vi "Check LVAddons Path List.vi"() -> ()   [LabVIEW 2023]
uses:
  <vilib>/Utility/Symbolic Paths/NI_SymbolicPaths.lvlib
  <vilib>/Utility/Symbolic Paths/Symbolic Path ID--enum.ctl
panel:
  out "all resolved paths":path[](array[path])
  # "Run this VI and verify that your LVAddon development location is in the list of paths.\n\nIf not, verify the correct paths are in the custom INI file and the .bat file that you used to launch LabVIEW."
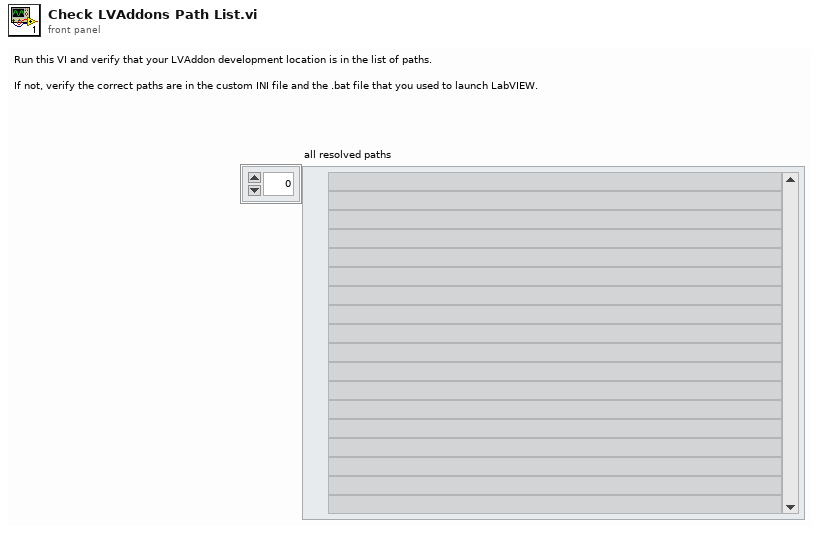
[diagram p1: front panel]
types:
  T1 = typedef "NI_SymbolicPaths.lvlib/Symbolic Path ID--enum.ctl" = enum16{"<invalid>", "<menus>", "<vilib>", "<userlib>", "<instrlib>", "<helpdir>", "<libdir>", "<osdatadir>", "<nishared>", "<instcachedir>", "<resource>", "<extravilib>"}
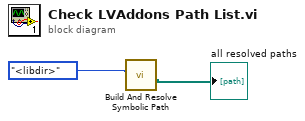
[diagram p0: block diagram]
diagram:
  n1 = call <vilib>:"Build And Resolve Symbolic Path.vi"("symbolic path id (<vilib>)"=Symbolic_Path_ID--enum."<libdir>") -> ("all resolved paths"=→"all resolved paths":path[])  [unwired: 8 in, 2 out]
